vi "KDH_4th_Ex3Task1.vi"() -> ()   [LabVIEW 2014, in "Harris_MacMaster_4th_LEGORobotics_11-29-16.lvrbt"]
uses:
  Harris_MacMaster_4th_LEGORobotics_11-29-16.lvrbt
  <vilib>/NXT/Dual Mode Library/Sensors/EV3_Ultrasonic_CM.vi
panel:
  in  "Stop Button":bool
  out "Distance LED":bool
  out "Wall Proximity":string
  in  "Min Distance":dbl
  in  "Max Distance":dbl
  out "Current Distance":dbl
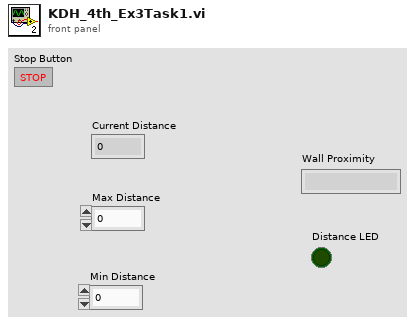
[diagram p1: front panel]
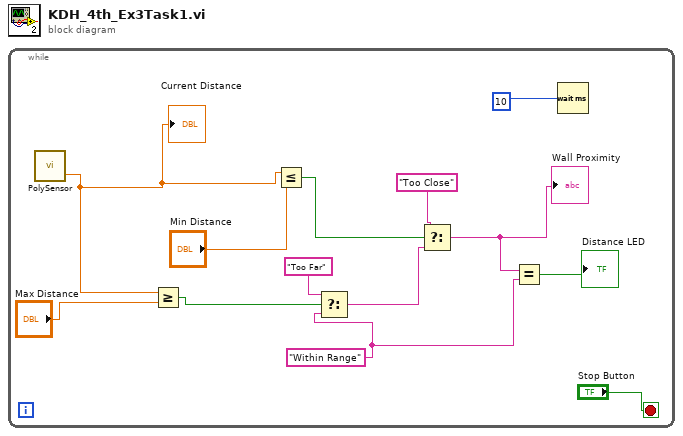
[diagram p0: block diagram]
diagram:
  n1 = while {
    stop <- "Stop Button" stop-if-true
    w4 = "Within Range"
    n2 = call-poly <vilib>:"PolySensor.vi"() -> ("Centimeters"=w9:sgl)  [unwired: 3 in, 1 out]
    "Current Distance" <- w9
    n3 = Greater Or Equal?(x=w9, y="Max Distance") -> (x >= y?=w12:bool)
    n4 = Less Or Equal?(x=w9, y="Min Distance") -> (x <= y?=w7:bool)
    n5 = Select(t="Too Far", s=w12, f=w4) -> (s? t:f=w6:string)
    n6 = Select(t="Too Close", s=w7, f=w6) -> (s? t:f=w3:string)
    "Wall Proximity" <- w3
    n7 = Equal?(x=w3, y=w4) -> (x = y?=→"Distance LED":bool)
    n8 = Wait (ms)(milliseconds to wait=u32 10 ("millisecond timer value")) -> ()  [unwired: 1 out]
  }
